vi "Motor Controller Write EEPROM.vi"(0 "COM port":refnum<visa-resource-name>, 5 "RS-485 addr.":u8, 7 "EEPROM":T1={"N bits"=13, "dt (s)"=0.002, "Kp (/rpm)"=0.002, "Ti (s)"=0.015, "Td (s)"=0.0, "N bits_soft"=15, "dt_soft (s)"=0.002, "Kp_soft (/rpm)"=0.0005, "Ti_soft (s)"=2.5, "Td_soft (s)"=0.0, "Encoder counting edges"=4, "Encoder PPR"=256, "Final drive ratio (X:1)"=4.071429, "Current zero offset (A)"=0.0, "RS-485 address"=1, "RS-485 baud rate"=500000, "Data output period (us)"=10000, "RPM setpoint"=0.0, "USB streaming enabled"=FALSE, "Operating mode"=3, "Running mode"=1, "EEPROM CRC-16"=29801} {"Running mode" items=["NORMAL", "SOFT"]; "Operating mode" items=["RUN", "COAST", "BRAKE", "SLEEP"]; "EEPROM CRC-16" format="%04x"; "N bits_soft" min=8 max=16 step=1; "Td_soft (s)" format="%#_6f"; "Ti_soft (s)" format="%#_6f"; "Kp_soft (/rpm)" format="%#_6f"; "dt_soft (s)" format="%#_6f"; "N bits" min=8 max=16 step=1; "Td (s)" format="%#_6f"; "Ti (s)" format="%#_6f"; "Kp (/rpm)" format="%#_6f"; "dt (s)" format="%#_6f"}, 9 "Close port after action":bool=TRUE) -> (4 "COM port out":refnum<visa-resource-name>, 15 "Error out":errorcluster)   [LabVIEW 2020]
uses:
  ctls/CTRL_EEPROM.ctl
  ctls/CTRL_Cmd.ctl
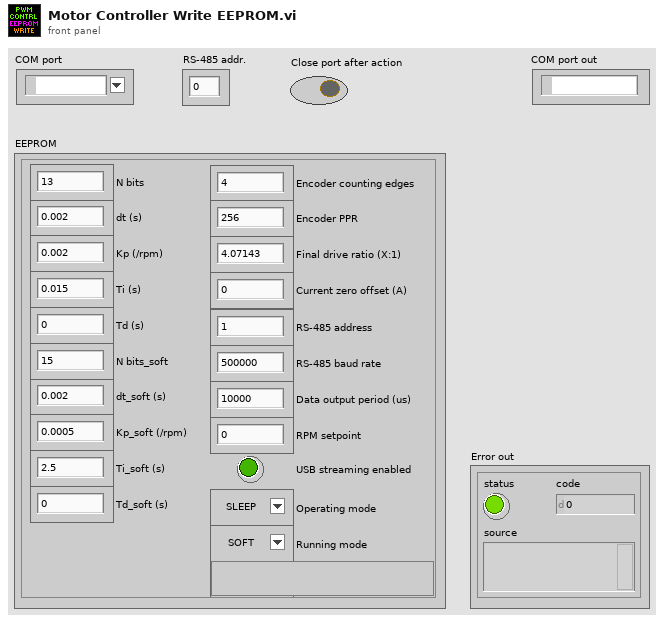
[diagram p1: front panel]
types:
  T1 = typedef "CTRL_EEPROM.ctl" = cluster{"N bits":u8, "dt (s)":sgl, "Kp (/rpm)":sgl, "Ti (s)":sgl, "Td (s)":sgl, "N bits_soft":u8, "dt_soft (s)":sgl, "Kp_soft (/rpm)":sgl, "Ti_soft (s)":sgl, "Td_soft (s)":sgl, "Encoder counting edges":u8, "Encoder PPR":u16, "Final drive ratio (X:1)":sgl, "Current zero offset (A)":sgl, "RS-485 address":u8, "RS-485 baud rate":u32, "Data output period (us)":u32, "RPM setpoint":sgl, "USB streaming enabled":bool, "Operating mode":u8, "Running mode":u8, "EEPROM CRC-16":u16}
  T2 = typedef "CTRL_Cmd.ctl" = string
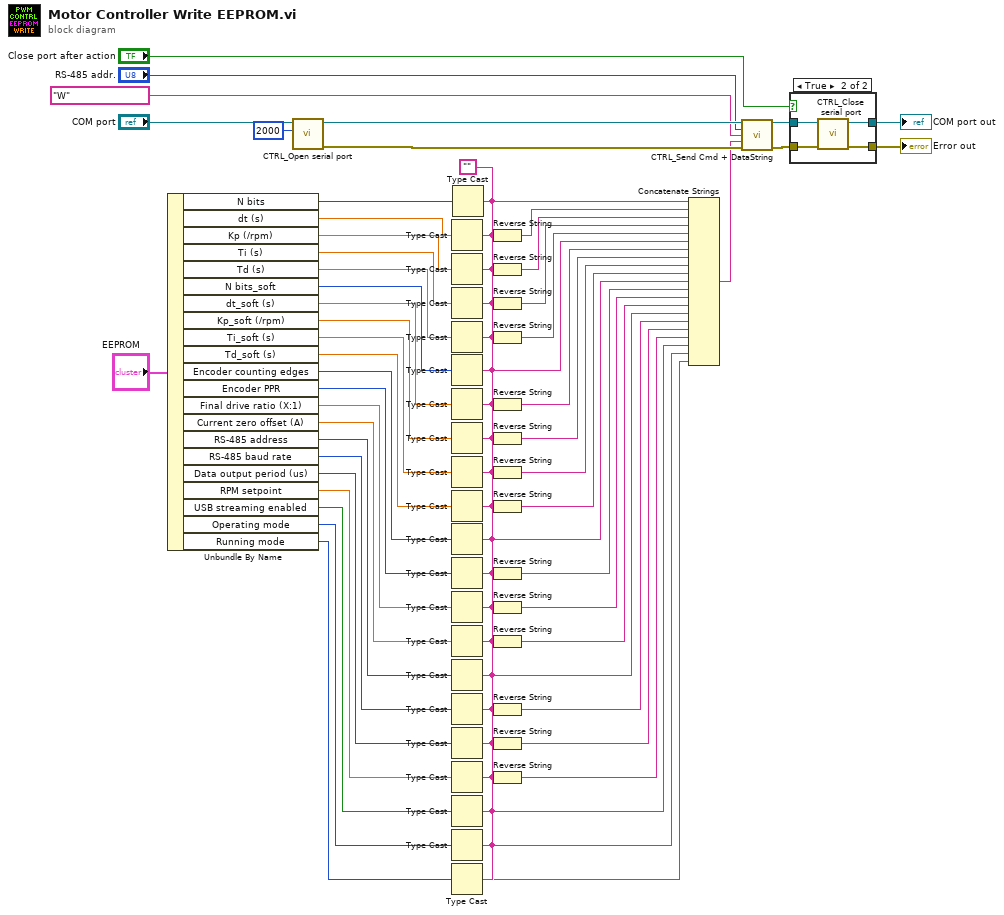
[diagram p0: block diagram]
diagram:
  w6 = ""
  n1 = Unbundle By Name("EEPROM") -> ("N bits"=w56:u8, "dt (s)"=w55:sgl, "Kp (/rpm)"=w54:sgl, "Ti (s)"=w51:sgl, "Td (s)"=w50:sgl, "N bits_soft"=w47:u8, "dt_soft (s)"=w41:sgl, "Kp_soft (/rpm)"=w40:sgl, "Ti_soft (s)"=w39:sgl, "Td_soft (s)"=w38:sgl, "Encoder counting edges"=w33:u8, "Encoder PPR"=w28:u16, "Final drive ratio (X:1)"=w26:sgl, "Current zero offset (A)"=w24:sgl, "RS-485 address"=w22:u8, "RS-485 baud rate"=w18:u32, "Data output period (us)"=w16:u32, "RPM setpoint"=w12:sgl, "USB streaming enabled"=w11:bool, "Operating mode"=w8:u8, "Running mode"=w7:u8)
  n2 = call "CTRL_Open serial port.vi"("timeout (ms)"=u32 2000, "VISA resource name"="COM port") -> ("Error out"=w67:errorcluster, "VISA resource name out"=w68:refnum<visa-resource-name>)  [unwired: 8 in]
  n3 = Type Cast(type=w6, x=w55) -> (*(type *) &x=w63:string)
  n4 = Type Cast(type=w6, x=w54) -> (*(type *) &x=w62:string)
  n5 = Type Cast(type=w6, x=w51) -> (*(type *) &x=w52:string)
  n6 = Type Cast(type=w6, x=w50) -> (*(type *) &x=w53:string)
  n7 = Type Cast(type=w6, x=w47) -> (*(type *) &x=w46:string)
  n8 = Type Cast(type=w6, x=w41) -> (*(type *) &x=w42:string)
  n9 = Type Cast(type=w6, x=w40) -> (*(type *) &x=w43:string)
  n10 = Type Cast(type=w6, x=w39) -> (*(type *) &x=w45:string)
  n11 = Type Cast(type=w6, x=w38) -> (*(type *) &x=w44:string)
  n12 = Type Cast(type=w6, x=w33) -> (*(type *) &x=w32:string)
  n13 = Type Cast(type=w6, x=w28) -> (*(type *) &x=w31:string)
  n14 = Type Cast(type=w6, x=w26) -> (*(type *) &x=w30:string)
  n15 = Type Cast(type=w6, x=w24) -> (*(type *) &x=w29:string)
  n16 = Type Cast(type=w6, x=w22) -> (*(type *) &x=w21:string)
  n17 = Type Cast(type=w6, x=w18) -> (*(type *) &x=w19:string)
  n18 = Type Cast(type=w6, x=w16) -> (*(type *) &x=w20:string)
  n19 = Type Cast(type=w6, x=w12) -> (*(type *) &x=w13:string)
  n20 = Type Cast(type=w6, x=w11) -> (*(type *) &x=w9:string)
  n21 = Type Cast(type=w6, x=w8) -> (*(type *) &x=w5:string)
  n22 = Type Cast(type=w6, x=w7) -> (*(type *) &x=w4:string)
  n23 = Type Cast(type=w6, x=w56) -> (*(type *) &x=w59:string)
  n24 = Reverse String(1:w63) -> (0:w61:string)
  n25 = Reverse String(1:w62) -> (0:w60:string)
  n26 = Reverse String(1:w52) -> (0:w49:string)
  n27 = Reverse String(1:w53) -> (0:w48:string)
  n28 = Reverse String(1:w42) -> (0:w37:string)
  n29 = Reverse String(1:w43) -> (0:w36:string)
  n30 = Reverse String(1:w45) -> (0:w35:string)
  n31 = Reverse String(1:w44) -> (0:w34:string)
  n32 = Reverse String(1:w31) -> (0:w27:string)
  n33 = Reverse String(1:w30) -> (0:w25:string)
  n34 = Reverse String(1:w29) -> (0:w23:string)
  n35 = Reverse String(1:w19) -> (0:w17:string)
  n36 = Reverse String(1:w20) -> (0:w15:string)
  n37 = Reverse String(1:w13) -> (0:w10:string)
  n38 = Concatenate Strings(w59, w61, w60, w49, w48, w46, w37, w36, w35, w34, w32, w27, w25, w23, w21, w17, w15, w10, w9, w5, w4) -> (w2:string)
  n39 = call "CTRL_Send Cmd + DataString.vi"("Port"=w68, "RS-485 addr."="RS-485 addr.", "Cmd"=T2 "W", "DataString"=w2, "Error In"=w67) -> ("Port out"=w65:refnum<visa-resource-name>, "Error Out"=w64:errorcluster)  [unwired: 9 in]
  n40 = case shown="True" "Close port after action" {
    tunnel: [w72 w75] -> w66
    tunnel: w65 -> [w71 w73]
    tunnel: w64 -> [w72 w74]
    tunnel: [w71 w73] -> w1
    frame False {
    }
    frame True {
      n41 = call "CTRL_Close serial port.vi"("Error in"=w74, "VISA resource name"=w73) -> ("Error out"=w75:errorcluster)  [unwired: 9 in]
    }
  }
  "Error out" <- w66
  "COM port out" <- w1
